vi "E870_SetChannelValue.vi"(6 "Channel #":i32, 8 "error in (no error)":errorcluster, 10 "# Steps":dbl, 11 "System no.":i32) -> ()   [LabVIEW 2011]
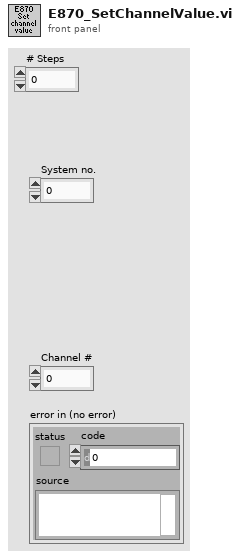
[diagram p1: front panel]
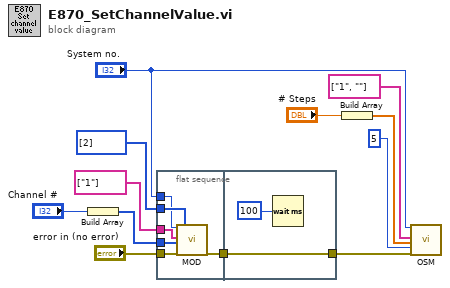
[diagram p0: block diagram]
diagram:
  n1 = Build Array("Channel #") -> (w2:i32[])
  n2 = flat-sequence {
    tunnel: w2 -> [w13]
    tunnel: "System no." -> [w14]
    tunnel: string[] ["1"] ("ItemID") -> [w15]
    tunnel: i32[] [2] ("Mode ID") -> [w16]
    tunnel: "error in (no error)" -> [w17]
    tunnel: [w18] -> w1
    tunnel: [w20] -> w7
    tunnel: w1 -> [w20]
    frame #0 {
      n3 = call "MOD.vi"("System no."=w14, "ItemID"=w15, "Value"=w13, "error in"=w17, "Mode ID"=w16) -> ("error out"=w18:errorcluster)  [unwired: 13 in, 1 out]
    }
    frame #1 {
      n4 = Wait (ms)(milliseconds to wait=u32 100) -> ()  [unwired: 1 out]
    }
  }
  n5 = Build Array("# Steps") -> (w4:dbl[])
  n6 = call "OSM.vi"("System no."="System no.", "Affected channels"=string[] ["1", ""], "No. of steps"=w4, "No.of digits"=i16 5, "error in"=w7) -> ()  [unwired: 14 in, 1 out]
